vi "Number to Proper Engl Text__ogtk.vi"(5 "Numeric":ext) -> (1 "String":string)   [LabVIEW 2011]
doc: "Converts a number to proper English text. Rounds off to whole numbers and can handle up to 10^63 (vigintillion) places."
panel:
  out "hasOnesPlace":bool
  out "isTeen":bool
  out "hasTensPlace":bool
  out "hasHundredsPlace":bool
  # "[OpenG VI Tags] ***Do Not Remove***"
  # "Number to Proper English Text.vi\n\nConverts an integer to proper English text.\n\nPlease visit http://www.OpenG.org to learn about the\nOpen Source LabVIEW software movement.\n\nNOTICE -- YOU MUST LEAVE THIS NOTICE IN PLACE.  PER THE TERMS OF THE LICENSE BELOW, YOU MAY SUBLICENSE THIS SOFTWARE \nIN ANY WAY THAT DOES NOT CONFLICT WITH THIS LICENSE.\n\n### BSD License (http://www.opensource.org/licenses/bsd-license.php) Begin ###\n \nCopyright (c) 2002, Jim Kring <jim@jimkring.com>\n\nAll rights reserved.\n\nRedistribution and use in source and binary forms, with or without modification, are permitted provided that the following conditions are met:\n\n    * Redistributions of source code must retain the above copyright notice, this list of conditions and the following disclaimer.\n    * Redistributions in binary form must reproduce the above copyright notice, this list of conditions and the following disclaimer in the \n       documentation and/or other materials provided with the distribution.\n    * Neither the name of SciWare, James Kring, Inc., nor the names of its contributors may be used to endorse or promote products derived \n       from this software without specific prior written permission.\n\nTHIS SOFTWARE IS PROVIDED BY THE COPYRIGHT HOLDERS AND CONTRIBUTORS \"AS IS\" AND ANY EXPRESS OR IMPLIED WARRANTIES, \nINCLUDING, BUT NOT LIMITED TO, THE IMPLIED WARRANTIES OF MERCHANTABILITY AND FITNESS FOR A PARTICULAR PURPOSE ARE \nDISCLAIMED. IN NO EVENT SHALL THE COPYRIGHT OWNER OR CONTRIBUTORS BE LIABLE FOR ANY DIRECT, INDIRECT, INCIDENTAL,\n SPECIAL, EXEMPLARY, OR CONSEQUENTIAL DAMAGES (INCLUDING, BUT NOT LIMITED TO, PROCUREMENT OF SUBSTITUTE GOODS OR \nSERVICES; LOSS OF USE, DATA, OR PROFITS; OR BUSINESS INTERRUPTION) HOWEVER CAUSED AND ON ANY THEORY OF LIABILITY, \nWHETHER IN CONTRACT, STRICT LIABILITY, OR TORT (INCLUDING NEGLIGENCE OR OTHERWISE) ARISING IN ANY WAY OUT OF THE USE \nOF THIS SOFTWARE, EVEN IF ADVISED OF THE POSSIBILITY OF SUCH DAMAGE.\n\n### BSD License End ###"
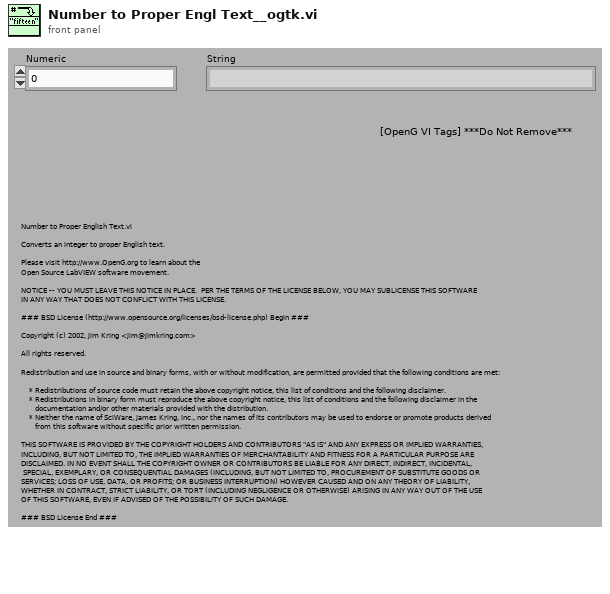
[diagram p1: front panel]
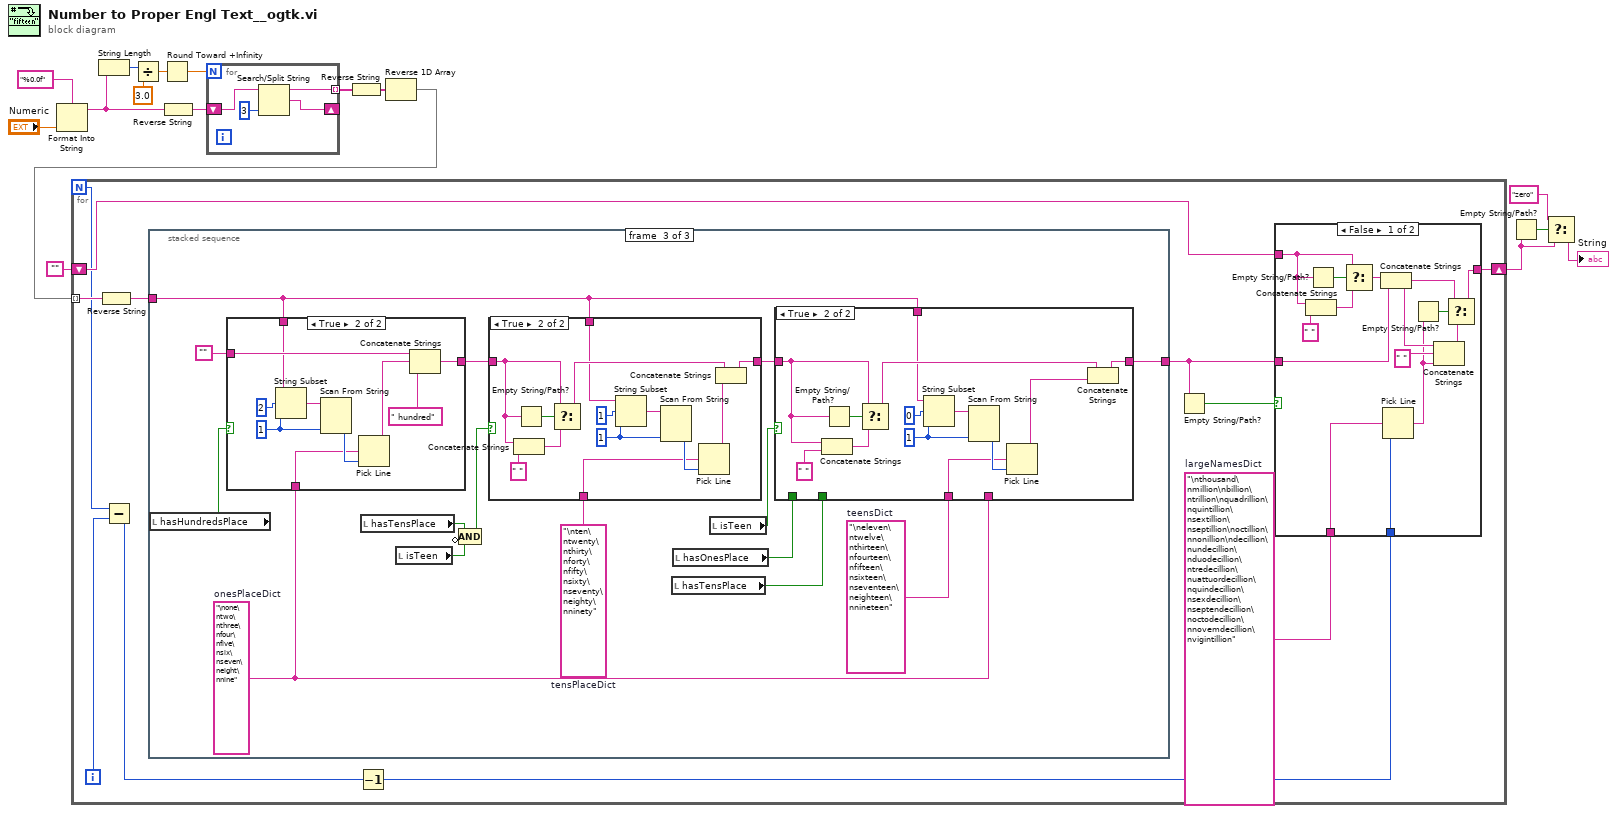
[diagram p0: block diagram]
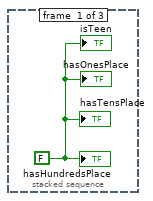
[diagram p3: hidden frame]
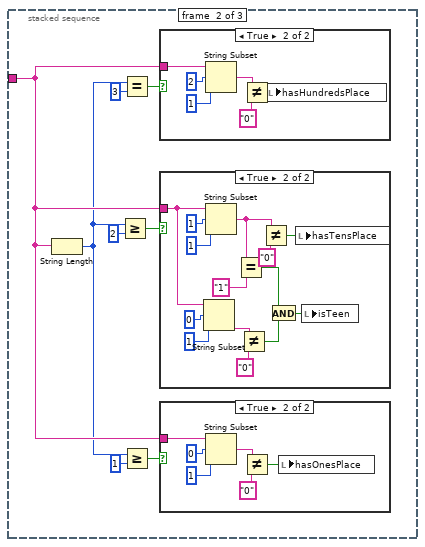
[diagram p4: hidden frame]
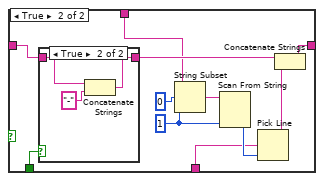
[diagram p9: hidden frame]
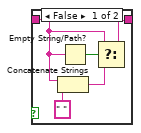
[diagram p10: hidden frame]
diagram:
  n1 = Format Into String(format string="%0.0f" ("Format String"), "Numeric") -> (resulting string=w11:string)  [unwired: 2 in, 1 out]
  n2 = String Length(string=w11) -> (length=w14:i32)
  n3 = Divide(x=w14, y=3.0) -> (x/y=w13:dbl)
  n4 = Round Toward +Infinity(x=w13) -> (ceil(x): smallest int >= x=w12:dbl)
  n5 = Reverse String(1:w11) -> (0:w10:string)
  n6 = for {
    N: w12 -> [_]
    shift-right: [w18] -> _
    shift-left: w10 -> [w20]
    tunnel: [w17] -> w9 mode=indexing
    n7 = Search/Split String(string=w20, offset (0)=3) -> (substring before match=w17:string, match + rest of string=w18:string)  [unwired: 1 in, 1 out]
  }
  n8 = Reverse String(1:w9) -> (0:w7:string[])
  n9 = Reverse 1D Array(array=w7) -> (reversed array=w6:string[])
  n10 = for {
    N -> [w25]
    shift-right: [w26] -> w3
    shift-left: "" -> [w27]
    tunnel: w6 -> [w30] mode=indexing
    i -> [w23]
    w21 = "\nthousand\nmillion\nbillion\ntrillion\nquadrillion\nquintillion\nsextillion\nseptillion\noctillion\nnonillion\ndecillion\nundecillion\nduodecillion\ntredecillion\nuattuordecillion\nquindecillion\nsexdecillion\nseptendecillion\noctodecillion\nnovemdecillion\nvigintillion"  # largeNamesDict
    n11 = Reverse String(1:w30) -> (0:w31:string)
    n12 = Subtract(x=w25, y=w23) -> (x-y=w24:i32)
    n13 = stacked-sequence {
      tunnel: w31 -> [_ w49 w85]
      tunnel: [_ _ w86] -> w28
      frame #0 {
        w47 = FALSE
        "hasOnesPlace" <- w47
        "isTeen" <- w47
        "hasTensPlace" <- w47
        "hasHundredsPlace" <- w47
      }
      frame #1 {
        n14 = String Length(string=w49) -> (length=w48:i32)
        n15 = Greater Or Equal?(x=w48, y=2) -> (x >= y?=w52:bool)
        n16 = Equal?(x=w48, y=3) -> (x = y?=w54:bool)
        n17 = Greater Or Equal?(x=w48, y=1) -> (x >= y?=w51:bool)
        n18 = case shown="True" w54 {
          tunnel: w49 -> [_ w76]
          frame False {
          }
          frame True {
            n19 = String Subset(string=w76, offset (0)=2, length (rest)=1 ("length (rest)")) -> (substring=w79:string)
            n20 = Not Equal?(x=w79, y="0") -> (x != y?=w81:bool)
            n21 = local write "hasHundredsPlace"(w81) -> ()
          }
        }
        n22 = case shown="True" w52 {
          tunnel: w49 -> [_ w71]
          frame False {
          }
          frame True {
            n23 = String Subset(string=w71, offset (0)=0, length (rest)=1 ("length (rest)")) -> (substring=w69:string)
            n24 = String Subset(string=w71, offset (0)=1, length (rest)=1 ("length (rest)")) -> (substring=w67:string)
            n25 = Equal?(x=w67, y="1") -> (x = y?=w66:bool)
            n26 = Not Equal?(x=w69, y="0") -> (x != y?=w68:bool)
            n27 = Not Equal?(x=w67, y="0") -> (x != y?=w65:bool)
            n28 = And(x=w66, y=w68) -> (x .and. y?=w64:bool)
            n29 = local write "hasTensPlace"(w65) -> ()
            n30 = local write "isTeen"(w64) -> ()
          }
        }
        n31 = case shown="True" w51 {
          tunnel: w49 -> [_ w56]
          frame False {
          }
          frame True {
            n32 = String Subset(string=w56, offset (0)=0, length (rest)=1 ("length (rest)")) -> (substring=w59:string)
            n33 = Not Equal?(x=w59, y="0") -> (x != y?=w61:bool)
            n34 = local write "hasOnesPlace"(w61) -> ()
          }
        }
      }
      frame #2 {
        w82 = "\neleven\ntwelve\nthirteen\nfourteen\nfifteen\nsixteen\nseventeen\neighteen\nnineteen"  # teensDict
        w83 = "\nten\ntwenty\nthirty\nforty\nfifty\nsixty\nseventy\neighty\nninety"  # tensPlaceDict
        w84 = "\none\ntwo\nthree\nfour\nfive\nsix\nseven\neight\nnine"  # onesPlaceDict
        n35 = local read "hasHundredsPlace"() -> (w96:bool)
        n36 = case shown="True" w96 {
          tunnel: "" -> [w150 w153]
          tunnel: [w150 w154] -> w91
          tunnel: w85 -> [_ w152]
          tunnel: w84 -> [_ w151]
          frame False {
          }
          frame True {
            w158 = 1 ("length (rest)")
            n37 = String Subset(string=w152, offset (0)=2, length (rest)=w158) -> (substring=w159:string)
            n38 = Scan From String(input string=w159, default 1=w158) -> (output 1=w157:i32)  [unwired: 3 in, 3 out]
            n39 = Pick Line(multi-line string=w151, line index=w157) -> (output string=w155:string)  [unwired: 1 in]
            n40 = Concatenate Strings(w153, w155, " hundred" ("Substring")) -> (w154:string)
          }
        }
        n41 = local read "hasTensPlace"() -> (w93:bool)
        n42 = local read "isTeen"() -> (w94:bool)
        n43 = Compound Arithmetic op=AND(w93, invert w94) -> (w92:bool)
        n44 = case shown="True" w92 {
          tunnel: w91 -> [w136 w139]
          tunnel: [w136 w141] -> w90
          tunnel: w85 -> [_ w138]
          tunnel: w83 -> [_ w137]
          frame False {
          }
          frame True {
            w145 = 1 ("length (rest)")
            n45 = Concatenate Strings(w139, " " ("Substring")) -> (w147:string)
            n46 = Empty String/Path?(string/path=w139) -> (empty?=w149:bool)
            n47 = Select(t=w139, s=w149, f=w147) -> (s? t:f=w140:string)
            n48 = String Subset(string=w138, offset (0)=1, length (rest)=w145) -> (substring=w144:string)
            n49 = Scan From String(input string=w144, default 1=w145) -> (output 1=w146:i32)  [unwired: 3 in, 3 out]
            n50 = Pick Line(multi-line string=w137, line index=w146) -> (output string=w142:string)  [unwired: 1 in]
            n51 = Concatenate Strings(w140, w142) -> (w141:string)
          }
        }
        n52 = local read "hasTensPlace"() -> (w87:bool)
        n53 = local read "hasOnesPlace"() -> (w88:bool)
        n54 = local read "isTeen"() -> (w89:bool)
        n55 = case shown="True" w89 {
          tunnel: w90 -> [w101 w125]
          tunnel: [w99 w127] -> w86
          tunnel: w88 -> [w102 _]
          tunnel: w87 -> [w100 _]
          tunnel: w85 -> [w98 w124]
          tunnel: w84 -> [w97 _]
          tunnel: w82 -> [_ w123]
          frame False {
            n56 = case shown="False" w102 {
              tunnel: w101 -> [w103 w113]
              tunnel: w100 -> [_ w114]
              tunnel: [w103 w106] -> w99
              tunnel: w98 -> [_ w105]
              tunnel: w97 -> [_ w104]
              frame False {
              }
              frame True {
                w111 = 1 ("length (rest)")
                n57 = case shown="True" w114 {
                  tunnel: w113 -> [w116 w122]
                  tunnel: [w115 w120] -> w107
                  frame False {
                    n58 = Concatenate Strings(w116, " " ("Substring")) -> (w119:string)
                    n59 = Empty String/Path?(string/path=w116) -> (empty?=w117:bool)
                    n60 = Select(t=w116, s=w117, f=w119) -> (s? t:f=w115:string)
                  }
                  frame True {
                    n61 = Concatenate Strings(w122, "-" ("Substring")) -> (w120:string)
                  }
                }
                n62 = String Subset(string=w105, offset (0)=0, length (rest)=w111) -> (substring=w110:string)
                n63 = Scan From String(input string=w110, default 1=w111) -> (output 1=w112:i32)  [unwired: 3 in, 3 out]
                n64 = Pick Line(multi-line string=w104, line index=w112) -> (output string=w108:string)  [unwired: 1 in]
                n65 = Concatenate Strings(w107, w108) -> (w106:string)
              }
            }
          }
          frame True {
            w131 = 1 ("length (rest)")
            n66 = Concatenate Strings(w125, " " ("Substring")) -> (w133:string)
            n67 = Empty String/Path?(string/path=w125) -> (empty?=w135:bool)
            n68 = Select(t=w125, s=w135, f=w133) -> (s? t:f=w126:string)
            n69 = String Subset(string=w124, offset (0)=0, length (rest)=w131) -> (substring=w130:string)
            n70 = Scan From String(input string=w130, default 1=w131) -> (output 1=w132:i32)  [unwired: 3 in, 3 out]
            n71 = Pick Line(multi-line string=w123, line index=w132) -> (output string=w128:string)  [unwired: 1 in]
            n72 = Concatenate Strings(w126, w128) -> (w127:string)
          }
        }
      }
    }
    n73 = Decrement(x=w24) -> (x-1=w22:i32)
    n74 = Empty String/Path?(string/path=w28) -> (empty?=w29:bool)
    n75 = case shown="False" w29 {
      tunnel: w28 -> [w40 _]
      tunnel: w27 -> [w42 w46]
      tunnel: [w38 w46] -> w26
      tunnel: w22 -> [w33 _]
      tunnel: w21 -> [w32 _]
      frame False {
        n76 = Concatenate Strings(w42, " " ("Substring")) -> (w43:string)
        n77 = Empty String/Path?(string/path=w42) -> (empty?=w45:bool)
        n78 = Select(t=w42, s=w45, f=w43) -> (s? t:f=w41:string)
        n79 = Concatenate Strings(w41, w40) -> (w36:string)
        n80 = Pick Line(multi-line string=w32, line index=w33) -> (output string=w35:string)  [unwired: 1 in]
        n81 = Empty String/Path?(string/path=w35) -> (empty?=w39:bool)
        n82 = Concatenate Strings(w36, " " ("Substring"), w35) -> (w34:string)
        n83 = Select(t=w36, s=w39, f=w34) -> (s? t:f=w38:string)
      }
      frame True {
      }
    }
  }
  n84 = Empty String/Path?(string/path=w3) -> (empty?=w4:bool)
  n85 = Select(t="zero", s=w4, f=w3) -> (s? t:f=→"String":string)
